vi "Record Data From Both Diodes.vi"() -> ()   [LabVIEW 2018]
uses:
  <vilib>/DAQmx/read.llb/DAQmx Read (Analog DBL 1Chan 1Samp).vi
  <vilib>/DAQmx/create/channels.llb/DAQmx Create Channel (AI-Voltage-Basic).vi
  <vilib>/DAQmx/miscellaneous.llb/DAQmx Fill In Error Info.vi
panel:
  in  "Other Diode":tag
  in  "stop":bool
  in  "Germanium Diode":tag
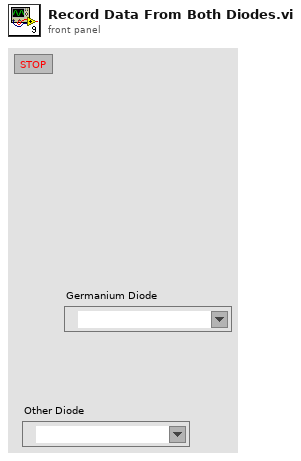
[diagram p1: front panel]
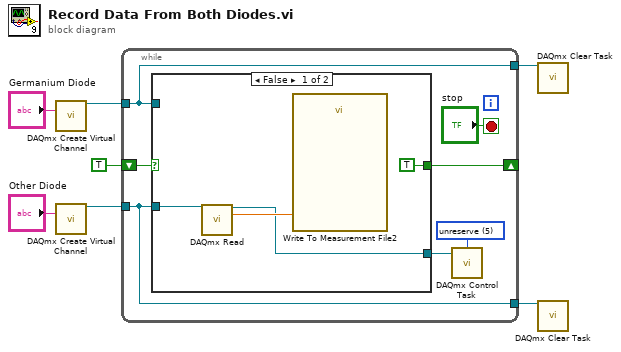
[diagram p0: block diagram]
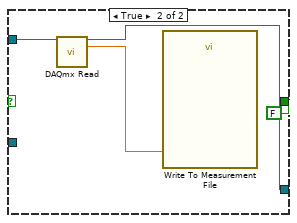
[diagram p2: hidden frame]
diagram:
  n1 = call-poly <vilib>:"DAQmx Create Virtual Channel.vi"("physical channels"="Germanium Diode") -> ("task out"=w6:refnum<k21>)  [unwired: 13 in, 1 out]
  n2 = call-poly <vilib>:"DAQmx Create Virtual Channel.vi"("physical channels"="Other Diode") -> ("task out"=w4:refnum<k21>)  [unwired: 13 in, 1 out]
  n3 = while {
    tunnel: w6 -> [w11]
    shift-right: [w13] -> _
    shift-left: TRUE -> [w12]
    tunnel: w4 -> [w10]
    tunnel: [w11] -> w2
    tunnel: [w10] -> w1
    stop <- "stop" stop-if-true
    w8 = 5 items=["verify"=2, "reserve"=4, "commit"=3, "unreserve"=5, "abort"=6] ("action")
    n4 = case shown="False" w12 {
      tunnel: w11 -> [_ w22]
      tunnel: [TRUE FALSE] -> w13
      tunnel: w10 -> [w17 _]
      tunnel: [w15 w19] -> w9
      frame False {
        n5 = call-poly <vilib>:"DAQmx Read.vi"("task/channels in"=w17) -> ("task out"=w15:refnum<k21>, "data"=w18:dbl)  [unwired: 12 in, 1 out]
        n6 = call "Write To Measurement File2"("Signals"=w18) -> ()  [unwired: 16 in, 3 out]
      }
      frame True {
        n7 = call-poly <vilib>:"DAQmx Read.vi"("task/channels in"=w22) -> ("task out"=w19:refnum<k21>, "data"=w21:dbl)  [unwired: 12 in, 1 out]
        n8 = call "Write To Measurement File"("Signals"=w21) -> ()  [unwired: 16 in, 3 out]
      }
    }
    n9 = call <vilib>:"DAQmx Control Task.vi"("task/channels in"=w9, "action"=w8) -> ()  [unwired: 12 in, 2 out]
  }
  n10 = call <vilib>:"DAQmx Clear Task.vi"("task in"=w2) -> ()  [unwired: 14 in, 1 out]
  n11 = call <vilib>:"DAQmx Clear Task.vi"("task in"=w1) -> ()  [unwired: 14 in, 1 out]
